vi "trash_Test Connection.vi"(8 "error in (no error)":errorcluster, 11 "CIF_UI in":refnum<class "CIF_UI.lvclass">) -> (0 "error out":errorcluster, 3 "CIF_UI out":refnum<class "CIF_UI.lvclass">)   [LabVIEW 2021]
uses:
  CIF_UI.lvclass
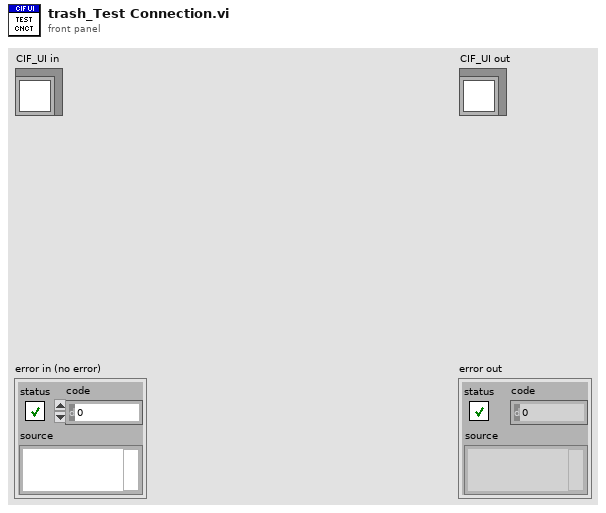
[diagram p1: front panel]
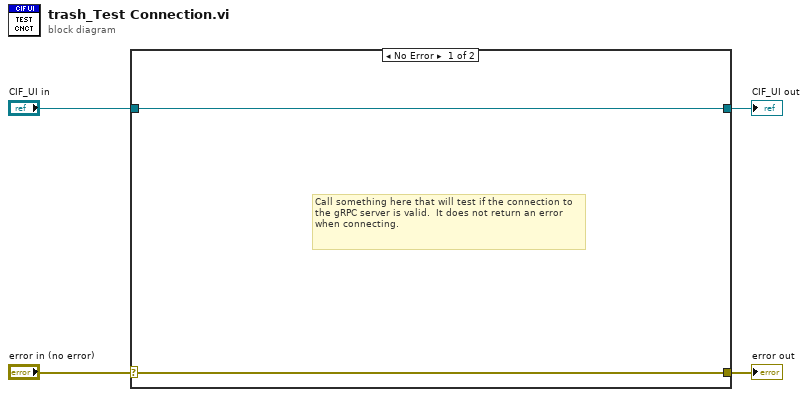
[diagram p0: block diagram]
diagram:
  n1 = case shown="No Error" "error in (no error)" {
    selector: "error in (no error)" -> [w5 w8]
    tunnel: [w5 w8] -> w3
    tunnel: [w6 w7] -> w1
    tunnel: "CIF_UI in" -> [w6 w7]
    frame No Error {
      # "Call something here that will test if the connection to the gRPC server is valid.  It does not return an error when connecting."
    }
    frame Error {
    }
  }
  "error out" <- w3
  "CIF_UI out" <- w1
